vi "LAB 7.vi"() -> ()   [LabVIEW 2022 SP3]
uses:
  <vilib>/Instr/_visa.llb/VISA Configure Serial Port (Instr).vi
panel:
  out "referencia":string
  in  "Knob":i16(knob) scale=250.0..330.0
  out "error":ext format="%.2f"
  out "sensor":string
  out "referencia":string
  out "señal de control":ext format="%.2f"
  out "temperatura 2":dbl(slide) scale=0.0..40.0
  out "error":dbl(knob) scale=-100.0..100.0
  in  "stop":bool
  out "referencia":dbl(slide) scale=0.0..40.0
  out "lectura de datos":string
  in  "puerto":refnum<visa-resource-name>
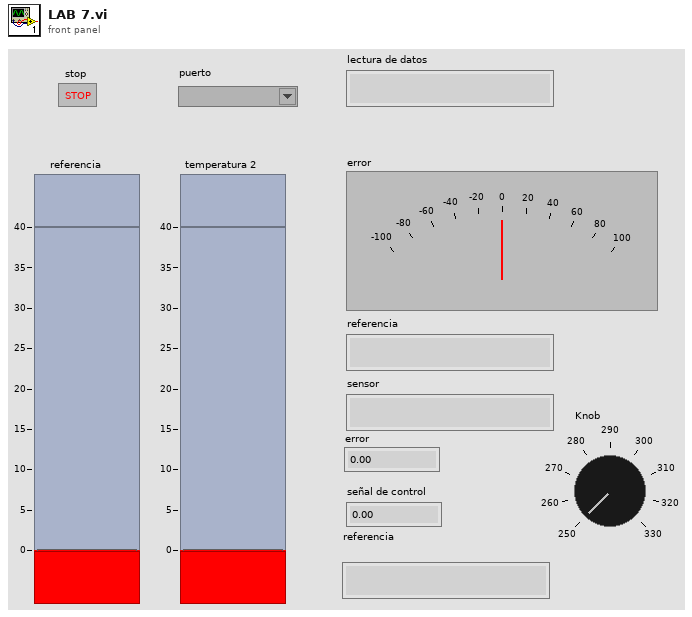
[diagram p1: front panel]
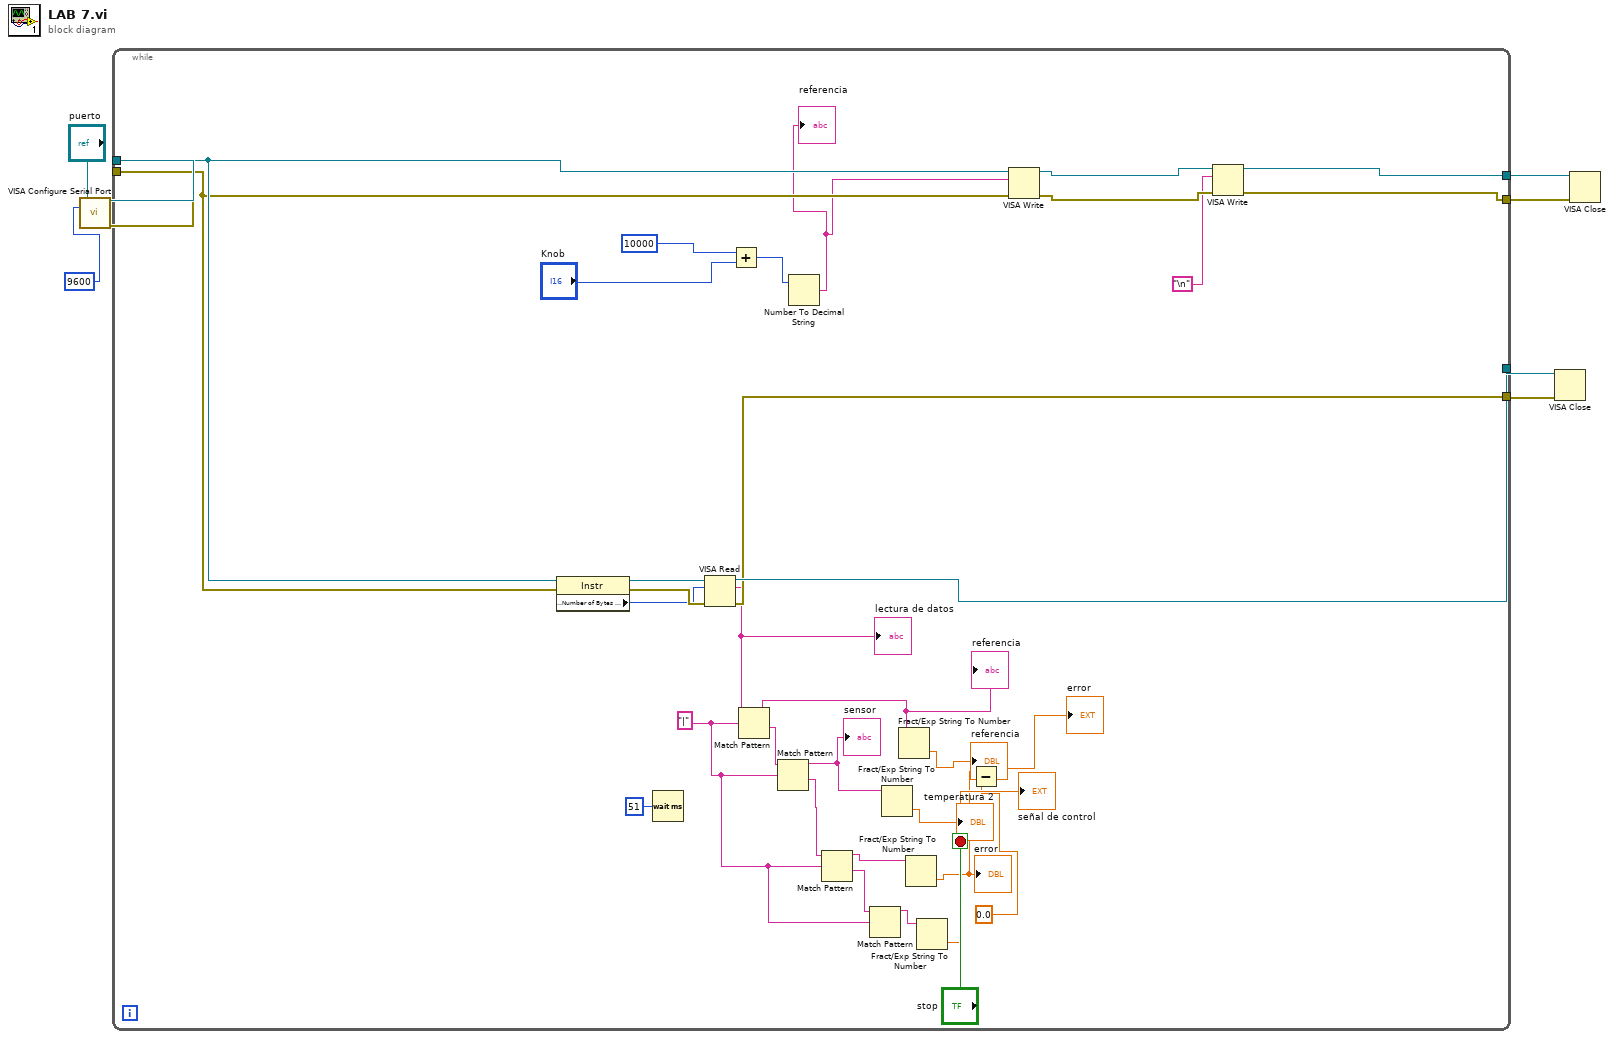
[diagram p0: block diagram]
diagram:
  n1 = call-poly "VISA Configure Serial Port"("VISA resource name"="puerto", "baud rate (9600)"=u32 9600) -> ("VISA resource name out"=w8:refnum<visa-resource-name>, "error out"=w6:errorcluster)  [unwired: 12 in]
  n2 = while {
    tunnel: w8 -> [w19]
    tunnel: [w36] -> w7
    tunnel: w6 -> [w18]
    tunnel: [w35] -> w5
    tunnel: [w14] -> w2
    tunnel: [w13] -> w1
    stop <- "stop" stop-if-true
    w30 = "|"
    n3 = property class="Instr"(reference=w19, error in=w18) -> (reference out=w41:refnum<visa-resource-name>, error out=w40:errorcluster, "Serial Settings:Number of Bytes at Serial Port"=w38:u32)
    n4 = Wait (ms)(milliseconds to wait=u32 51) -> ()  [unwired: 1 out]
    n5 = VISA Read(VISA resource name=w41, byte count=w38, error in (no error)=w40) -> (VISA resource name out=w36:refnum<visa-resource-name>, read buffer=w34:string, error out=w35:errorcluster)  [unwired: 1 out]
    "lectura de datos" <- w34
    n6 = Add(x=i16 10000, y="Knob") -> (x+y=w9:i16)
    n7 = Match Pattern(string=w34, regular expression=w30) -> (before substring=w26:string, after substring=w33:string)  [unwired: 1 in, 2 out]
    "referencia" <- w26
    n8 = Match Pattern(string=w33, regular expression=w30) -> (before substring=w25:string, after substring=w32:string)  [unwired: 1 in, 2 out]
    "sensor" <- w25
    n9 = Number To Decimal String(number=w9) -> (decimal integer string=w17:string)  [unwired: 1 in]
    "referencia" <- w17
    n10 = Match Pattern(string=w32, regular expression=w30) -> (before substring=w24:string, after substring=w31:string)  [unwired: 1 in, 2 out]
    n11 = Match Pattern(string=w31, regular expression=w30) -> (before substring=w23:string)  [unwired: 1 in, 3 out]
    n12 = Fract/Exp String To Number(string=w25) -> (number=→"temperatura 2":dbl)  [unwired: 3 in, 1 out]
    n13 = Fract/Exp String To Number(string=w26) -> (number=→"referencia":dbl)  [unwired: 3 in, 1 out]
    n14 = Fract/Exp String To Number(string=w24) -> (number=w20:dbl)  [unwired: 3 in, 1 out]
    "error" <- w20
    n15 = Fract/Exp String To Number(string=w23) -> (number=→"señal de control":dbl)  [unwired: 3 in, 1 out]
    n16 = Subtract(x=w20, y=0.0) -> (x-y=→"error":dbl)
    n17 = VISA Write(VISA resource name=w19, write buffer=w17, error in (no error)=w18) -> (VISA resource name out=w16:refnum<visa-resource-name>, error out=w15:errorcluster)  [unwired: 1 out]
    n18 = VISA Write(VISA resource name=w16, write buffer="\n", error in (no error)=w15) -> (VISA resource name out=w14:refnum<visa-resource-name>, error out=w13:errorcluster)  [unwired: 1 out]
  }
  n19 = VISA Close(VISA resource name=w7, error in (no error)=w5) -> ()  [unwired: 1 out]
  n20 = VISA Close(VISA resource name=w2, error in (no error)=w1) -> ()  [unwired: 1 out]
